vi "Connect.vi"(8 "error in (no error)":errorcluster, 10 "Channel(s)":string, 11 "Switch_Concrete in":refnum<class "Switch_Concrete.lvclass">) -> (0 "error out":errorcluster, 3 "Switch_Concrete out":refnum<class "Switch_Concrete.lvclass">)   [LabVIEW 2024, in "HAL_Example.lvlib" / "Switch_Concrete.lvclass"]
uses:
  Switch_Concrete.lvclass
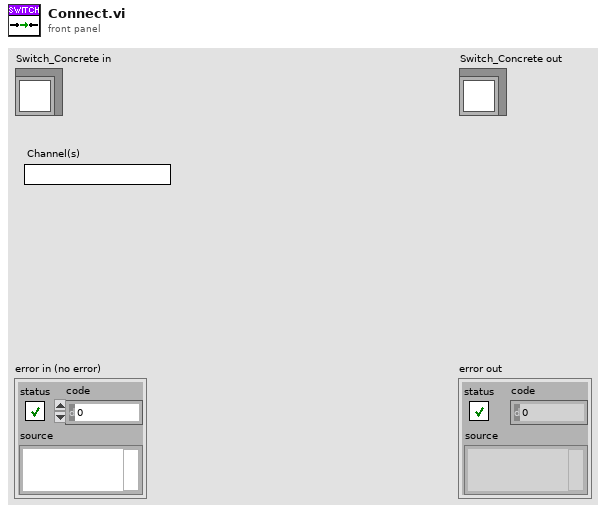
[diagram p1: front panel]
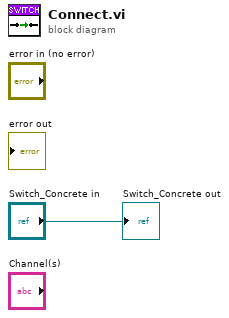
[diagram p0: block diagram]
diagram:
  "Switch_Concrete out" <- "Switch_Concrete in"
